vi "Sequence.SeperateMainSections.vi"(8 "error in (no error)":errorcluster, 10 "UI.Sequence#ofColumns":i32, 11 "MulticolumnListbox in":refnum<vi>) -> (0 "error out":errorcluster, 1 "Conditions":string[][](array[string]), 2 "Duration":string[](array[string]), 3 "Steps":string[][](array[string]))   [LabVIEW 2013, in "Simple Sequence Tools - Editor.lvlib"]
uses:
  Simple Sequence Tools - Editor.lvlib
  Shared/SubVIs/Main.Constants.vi
  Shared/Simple Sequence Tools - Shared.lvlib
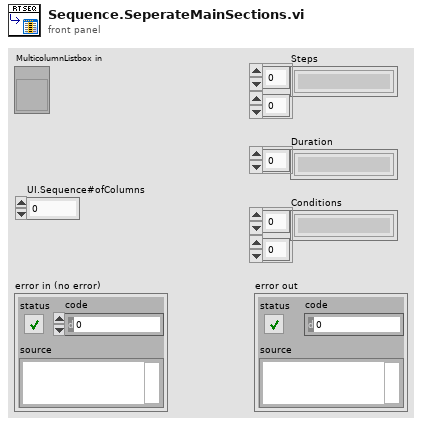
[diagram p1: front panel]
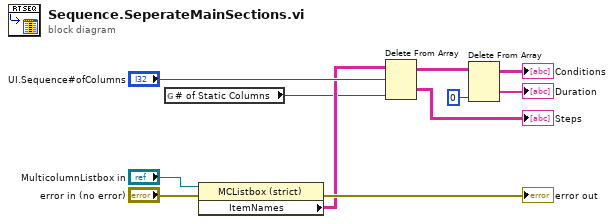
[diagram p0: block diagram]
diagram:
  n1 = global read "Main.Constants.vi" "# of Static Columns"() -> (w2:u32)
  n2 = property class="MCListbox (strict)"(reference="MulticolumnListbox in", error in="error in (no error)") -> (error out=→"error out":errorcluster, "ItemNames"=w4:string[][])  [unwired: 1 out]
  n3 = Delete From Array(array=w4, length="UI.Sequence#ofColumns", index (col)=w2) -> (deleted portion=→"Steps":string[][], array with subset deleted=w3:string[][])  [unwired: 1 in]
  n4 = Delete From Array(array=w3, index (col)=0 ("disabled index (col)")) -> (deleted portion=→"Duration":string[], array with subset deleted=→"Conditions":string[][])  [unwired: 2 in]
